vi "Pre Launch Init.vi"(11 "Nested in":refnum<class "Thermometer Multichannel Worker.lvclass">) -> (0 "error out":errorcluster, 3 "Nested out":refnum<class "Thermometer Multichannel Worker.lvclass">)   [LabVIEW 2024, in "Thermometer Multichannel Worker.lvlib" / "Thermometer Multichannel Worker.lvclass"]
doc: "(<B>Filename</B>: Actor Framework.lvlib:Actor.lvclass:Pre Launch Init.vi)\n\nDefines behavior that occurs after the Launch Nested Actor method is invoked but before the actor's Actor Core method begins running.\n\nBy default, this method does nothing. A descendant class may override it to define behavior."
uses:
  Thermometer Multichannel Worker.lvclass
  Interfaces/IConfigure/IConfigure.lvclass
  Thermometer Multichannel Worker.lvclass/Thermometer Multichannel Worker.ctl
  Interfaces/IRead Temperature Multichannel/IRead Temperature Multichannel.lvclass
  Interfaces/IConfiguration/IConfiguration.lvclass
  <vilib>/ActorFramework/Actor/Actor.lvclass
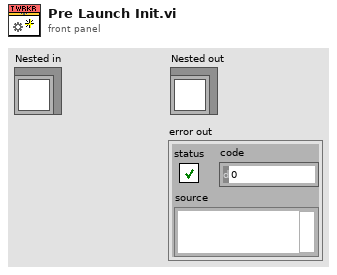
[diagram p1: front panel]
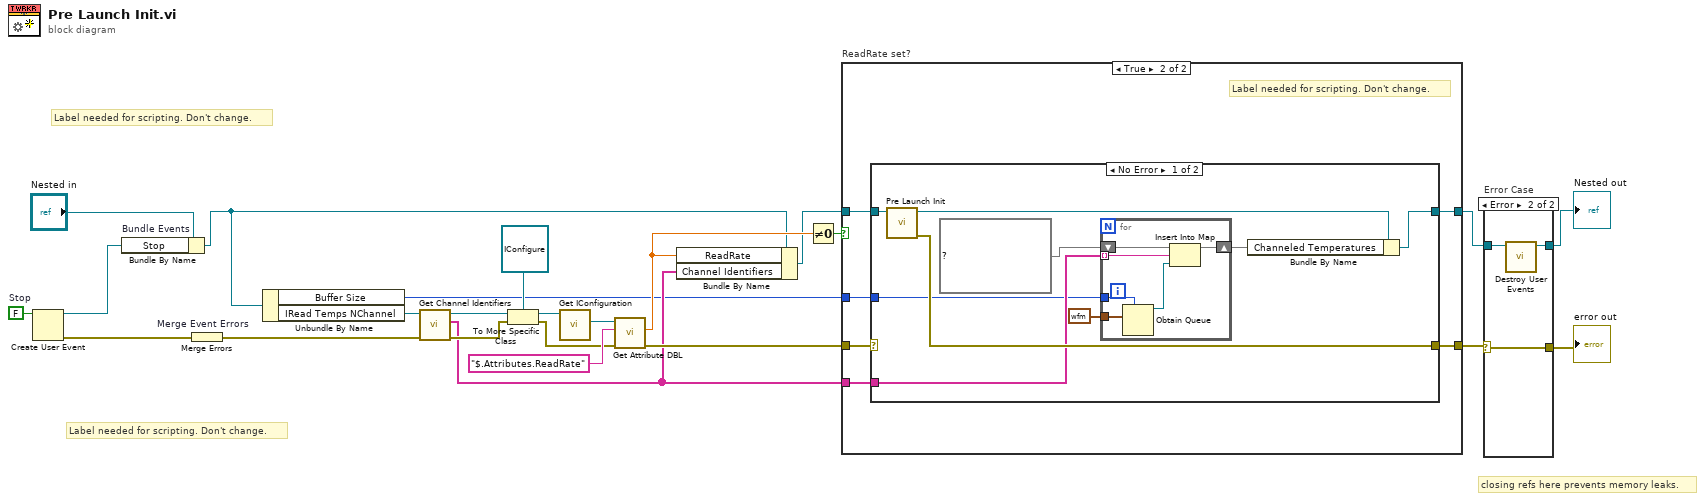
[diagram p0: block diagram]
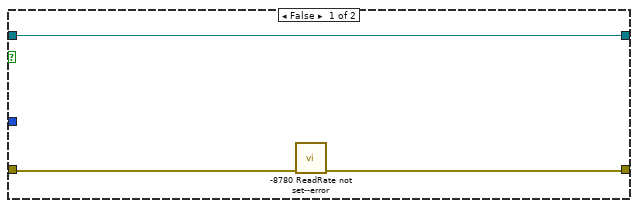
[diagram p2: hidden frame]
diagram:
  w10 = FALSE  # Stop
  # "closing refs here prevents memory leaks."
  # "Label needed for scripting. Don't change."
  # "Label needed for scripting. Don't change."
  n1 = Create User Event(user event datatype=w10) -> (user event=w8:refnum<user-event>, error out=w9:errorcluster)  [unwired: 1 in]
  n2 = Bundle By Name "Bundle Events"(cluster="Nested in", "Stop"=w8) -> (w6:refnum<class "Thermometer Multichannel Worker.lvclass">)
  n3 = Merge Errors "Merge Event Errors"(w9) -> (w5:errorcluster)
  n4 = Unbundle By Name(w6) -> ("Buffer Size"=w11:i32, "IRead Temps NChannel"=w16:refnum<class "IRead Temperature Multichannel.lvclass">)
  n5 = call-dynamic "Get Channel Identifiers.vi"("error in"=w5, "IRead Temperature Multichannel in"=w16) -> ("error out"=w14:errorcluster, "Channel Identifiers"=w12:string[], "IRead Temperature Multichannel out"=w15:refnum<class "IRead Temperature Multichannel.lvclass">)  [unwired: 7 in]
  n6 = To More Specific Class(target class=refnum<class "IConfigure.lvclass"> refnum ("IConfigure.lvclass"), reference=w15, error in=w14) -> (specific class reference=w22:refnum<class "IConfigure.lvclass">, error out=w19:errorcluster)
  n7 = call-dynamic "Get IConfiguration.vi"("IConfigure in"=w22) -> ("IConfiguration"=w21:refnum<class "IConfiguration.lvclass">)  [unwired: 9 in, 1 out]
  n8 = call-dynamic "Get Attribute DBL.vi"("error in"=w19, "Attribute"="$.Attributes.ReadRate", "IConfiguration in"=w21) -> ("error out"=w13:errorcluster, "Value"=w18:dbl)  [unwired: 6 in, 1 out]
  n9 = Bundle By Name(cluster=w6, "ReadRate"=w18, "Channel Identifiers"=w12) -> (w17:refnum<class "Thermometer Multichannel Worker.lvclass">)
  n10 = Not Equal To 0?(x=w18) -> (x != 0?=w24:bool)
  n11 = case "ReadRate set?" shown="True" w24 {
    tunnel: w17 -> [w27 w33]
    tunnel: w13 -> [w25 w32]
    tunnel: w12 -> [_ w31]
    tunnel: w11 -> [_ w30]
    tunnel: [w26 w29] -> w4
    tunnel: [w27 w28] -> w3
    frame False {
      n12 = call "-8780 ReadRate not set--error.vi"("error in"=w25) -> ("error out"=w26:errorcluster)  [unwired: 10 in]
    }
    frame True {
      # "Label needed for scripting. Don't change."
      n13 = case shown="No Error" w32 {
        selector: w32 -> [_ w50]
        tunnel: [w39 w49] -> w28
        tunnel: w33 -> [w42 w49]
        tunnel: [w41 w50] -> w29
        tunnel: w31 -> [w38 _]
        tunnel: w30 -> [w34 _]
        frame No Error {
          n14 = call-parent "Pre Launch Init.vi"("Actor in"=w42) -> ("error out"=w41:errorcluster, "Actor out"=w40:refnum<class "Thermometer Multichannel Worker.lvclass">)  [unwired: 9 in]
          n15 = for {
            tunnel: w38 -> [w47] mode=indexing
            shift-right: [w48] -> w37
            shift-left: map{string, refnum<queue>} {} ("Channeled Temperatures") -> [w46]
            tunnel: waveform(dbl) {"t0"=timestamp(0 s since 1904-01-01), "dt"=1.0, "Y"=[]} ("Waveform") -> [w45]
            tunnel: w34 -> [w43]
            n16 = Obtain Queue(max queue size (-1, unlimited)=w43, element data type=w45) -> (queue out=w44:refnum<queue>)  [unwired: 3 in, 2 out]
            n17 = Insert Into Map(map in=w46, key=w47, value=w44) -> (map out=w48:map{string, refnum<queue>})  [unwired: 2 out]
          }
          n18 = Bundle By Name(cluster=w40, "Channeled Temperatures"=w37) -> (w39:refnum<class "Thermometer Multichannel Worker.lvclass">)
        }
        frame Error {
        }
      }
    }
  }
  n19 = case "Error Case" shown="Error" w4 {
    selector: w4 -> [w51 w55]
    tunnel: w3 -> [w52 w54]
    tunnel: [w52 w53] -> w2
    tunnel: [w51 w55] -> w1
    frame No Error {
    }
    frame Error {
      n20 = call "Destroy User Events.vi"("UI Template in"=w54) -> ("UI Template out"=w53:refnum<class "Thermometer Multichannel Worker.lvclass">)  [unwired: 10 in]
    }
  }
  "error out" <- w1
  "Nested out" <- w2
